vi "LEP_RV_TestIfWriteObject.vi"(10 "Old decision":bool, 11 "Array of object's elements":string[](array[string])) -> (3 "Write ?":bool)   [LabVIEW 2011]
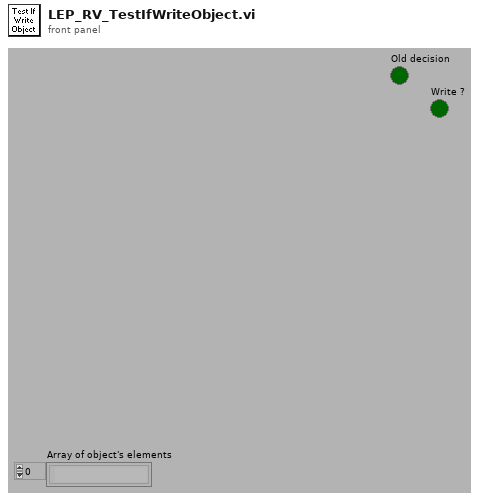
[diagram p1: front panel]
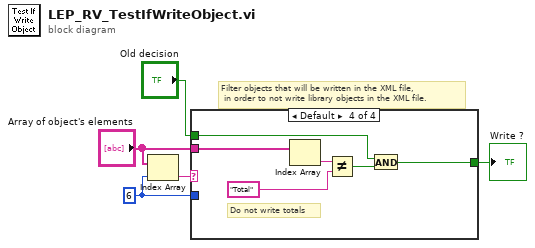
[diagram p0: block diagram]
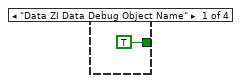
[diagram p2: hidden frame]
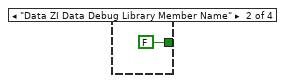
[diagram p3: hidden frame]
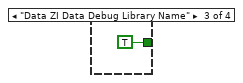
[diagram p4: hidden frame]
diagram:
  w2 = 6 ("index")
  # "Filter objects that will be written in the XML file,\n in order to not write library objects in the XML file."
  n1 = Index Array(array="Array of object's elements", index=w2) -> (element=w5:string)
  n2 = case shown="Default" w5 {
    tunnel: [TRUE ("Write ? 2") FALSE ("Write ? 2") TRUE ("Write ? 2") w9] -> w4
    tunnel: "Array of object's elements" -> [_ _ _ w14]
    tunnel: w2 -> [_ _ _ _]
    tunnel: "Old decision" -> [_ _ _ w11]
    frame "Data ZI Data Debug Object Name" {
    }
    frame "Data ZI Data Debug Library Member Name" {
    }
    frame "Data ZI Data Debug Library Name" {
    }
    frame Default {
      # "Do not write totals"
      n3 = Index Array(array=w14) -> (element=w13:string)  [unwired: 1 in]
      n4 = Not Equal?(x=w13, y="Total") -> (x != y?=w10:bool)
      n5 = And(x=w11, y=w10) -> (x .and. y?=w9:bool)
    }
  }
  "Write ?" <- w4
